vi "Data to Variant.vi"(10 "Value":string, 11 "Type":string) -> (0 "error out":errorcluster, 3 "Variant":variant)   [LabVIEW 2019, in "CAML.lvlib" / "CAML.lvclass"]
uses:
  <vilib>/gpm_packages/@cs/persistence/source/CAML/CAML.lvclass
  <vilib>/gpm_packages/@cs/data-type-serializer/source/Data Type/Data Type.lvclass
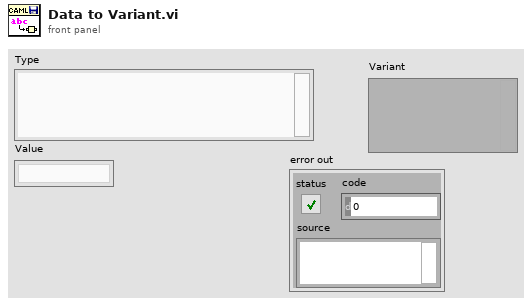
[diagram p1: front panel]
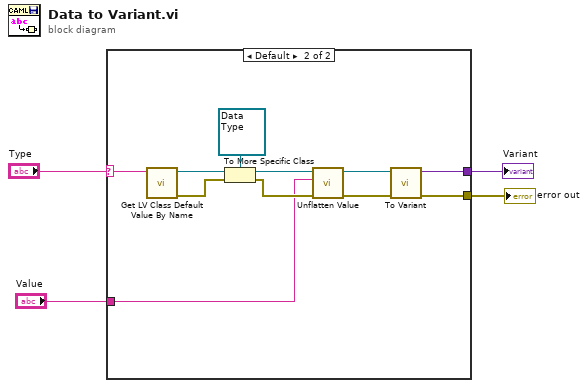
[diagram p0: block diagram]
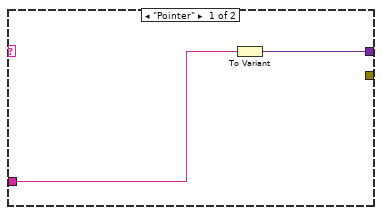
[diagram p2: hidden frame]
diagram:
  n1 = case shown="Default" "Type" {
    selector: "Type" -> [_ w10]
    tunnel: "Value" -> [w6 w9]
    tunnel: [w5 w8] -> w2
    tunnel: [_ w7] -> w1
    frame "Pointer" {
      n2 = To Variant(anything=w6) -> (Variant=w5:variant)
    }
    frame Default {
      n3 = call <vilib>:"Get LV Class Default Value By Name.vi"("class name"=w10) -> ("error out"=w15:errorcluster, "object"=w17:refnum<class>)  [unwired: 9 in]
      n4 = To More Specific Class(target class=refnum<class "Data Type.lvclass"> refnum ("Data Type.lvclass"), reference=w17, error in=w15) -> (specific class reference=w14:refnum<class "Data Type.lvclass">, error out=w12:errorcluster)
      n5 = call-dynamic "Unflatten Value.vi"("error in (no error)"=w12, "Value"=w9, "Data Type in"=w14) -> ("error out"=w11:errorcluster, "Data Type out"=w13:refnum<class "Data Type.lvclass">)  [unwired: 7 in]
      n6 = call-dynamic "To Variant.vi"("error in"=w11, "Data Type in"=w13) -> ("error out"=w7:errorcluster, "Variant"=w8:variant)  [unwired: 8 in]
    }
  }
  "Variant" <- w2
  "error out" <- w1
